vi "Generate Bitfile Path.vi"() -> (0 "Bitfile Path":path)   [LabVIEW 2019, in "Load And Parse Bitfile Testing.lvclass"]
uses:
  Load And Parse Bitfile Testing.lvclass
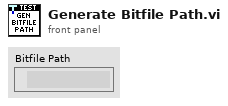
[diagram p1: front panel]
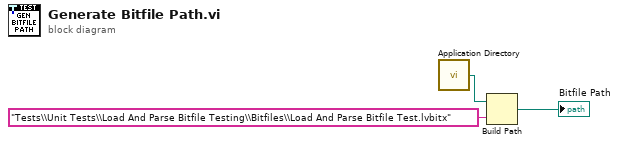
[diagram p0: block diagram]
diagram:
  n1 = call <vilib>:"Application Directory.vi"() -> ("Application Directory"=w2:path)
  n2 = Build Path(base path=w2, name or relative path="Tests\\Unit Tests\\Load And Parse Bitfile Testing\\Bitfiles\\Load And Parse Bitfile Test.lvbitx") -> (appended path=→"Bitfile Path":path)
